vi "string.RemoveIllegalChars.vi"(7 "mode (file)":enum16{"filename", "database", "alphanumeric"}(ring), 8 "error in (no error)":errorcluster, 11 "string in":string) -> (0 "error out":errorcluster, 2 "illegal characters":string, 3 "legal string out":string)   [LabVIEW 2020]
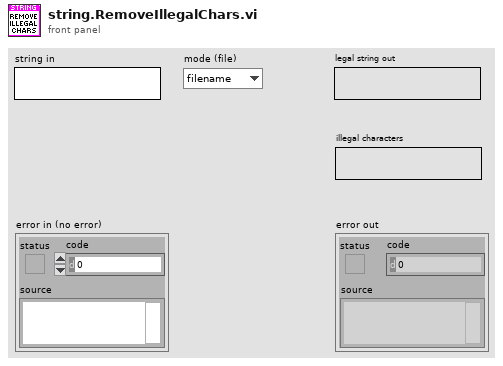
[diagram p1: front panel]
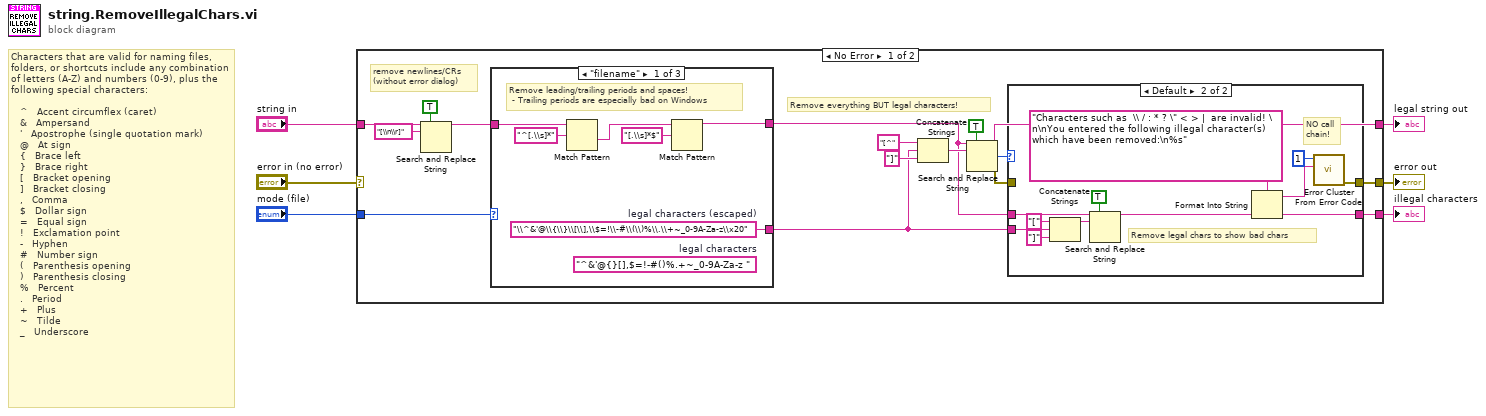
[diagram p0: block diagram]
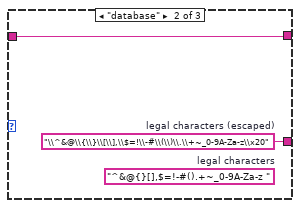
[diagram p2: hidden frame]
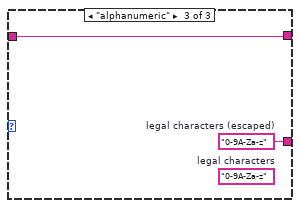
[diagram p3: hidden frame]
diagram:
  # "Characters that are valid for naming files, folders, or shortcuts include any combination of letters (A-Z) and numbers (0-9), plus the following special characters: \n\n   ^   Accent circumflex (caret)\n   &   Ampersand\n   '   Apostrophe (single quotation mark)\n   @   At sign\n   {   Brace left\n   }   Brace right\n   [   Bracket opening\n   ]   Bracket closing\n   ,   Comma\n   $   Dollar sign\n   =   Equal sign\n   !   Exclamation point\n   -   Hyphen\n   #   Number sign\n   (   Parenthesis opening\n   )   Parenthesis closing\n   %   Percent\n   .   Period\n   +   Plus\n   ~   Tilde\n   _   Underscore"
  n1 = case shown="No Error" "error in (no error)" {
    selector: "error in (no error)" -> [_ w45]
    tunnel: "string in" -> [w10 _]
    tunnel: [w21 _] -> w5
    tunnel: [w15 w45] -> w3
    tunnel: [w13 _] -> w2
    tunnel: "mode (file)" -> [w9 _]
    frame No Error {
      # "remove newlines/CRs\n(without error dialog)"
      # "Remove everything BUT legal characters!"
      n2 = Search and Replace String(replace all?=TRUE ("replace all? (F)"), input string=w10, search string="[\\n\\r]") -> (result string=w8:string)  [unwired: 5 in, 3 out]
      n3 = case shown="\"filename\"" w9 {
        tunnel: [w28 w30 w32] -> w17
        tunnel: w8 -> [w27 w29 w31]
        tunnel: [w23 w29 w31] -> w7
        frame "filename" {
          (unwired) "^&'@{}[],$=!-#()%.+~_0-9A-Za-z "  # legal characters
          w28 = "\\^&'@\\{\\}\\[\\],\\$=!\\-#\\(\\)%\\.\\+~_0-9A-Za-z\\x20"  # legal characters (escaped)
          # "Remove leading/trailing periods and spaces! \n - Trailing periods are especially bad on Windows"
          n4 = Match Pattern(string=w27, regular expression="^[.\\s]*") -> (after substring=w24:string)  [unwired: 1 in, 3 out]
          n5 = Match Pattern(string=w24, regular expression="[.\\s]*$") -> (before substring=w23:string)  [unwired: 1 in, 3 out]
        }
        frame "database" {
          (unwired) "^&@{}[],$=!-#().+~_0-9A-Za-z "  # legal characters
          w30 = "\\^&@\\{\\}\\[\\],\\$=!\\-#\\(\\)\\.\\+~_0-9A-Za-z\\x20"  # legal characters (escaped)
        }
        frame "alphanumeric" {
          (unwired) "0-9A-Za-z"  # legal characters
          w32 = "0-9A-Za-z"  # legal characters (escaped)
        }
      }
      n6 = Concatenate Strings("[^" ("string"), w17, "]" ("string")) -> (w20:string)
      n7 = Search and Replace String(replace all?=TRUE ("replace all? (F)"), input string=w7, search string=w20) -> (result string=w21:string, number of replacements=w14:i32, error out=w16:errorcluster)  [unwired: 5 in, 1 out]
      n8 = case shown="Default" w14 {
        tunnel: w17 -> [_ w44]
        tunnel: w16 -> [w33 _]
        tunnel: [w33 w34] -> w15
        tunnel: w7 -> [_ w41]
        tunnel: [_ w37] -> w13
        frame 0 {
          # "No bad chars!"
        }
        frame Default {
          # "NO call\nchain!"
          # "Remove legal chars to show bad chars"
          n9 = Concatenate Strings("[" ("string"), w44, "]" ("string")) -> (w40:string)
          n10 = Search and Replace String(replace all?=TRUE ("replace all? (F)"), input string=w41, search string=w40) -> (result string=w37:string)  [unwired: 5 in, 3 out]
          n11 = Format Into String(format string="Characters such as  \\ / : * ? \" < > |  are invalid! \n\nYou entered the following illegal character(s) which have been removed:\n%s", w37) -> (resulting string=w35:string)  [unwired: 2 in, 1 out]
          n12 = call <vilib>:"Error Cluster From Error Code.vi"("error message (\"\")"=w35, "error code (0)"=1) -> ("error out"=w34:errorcluster)  [unwired: 7 in]
        }
      }
    }
    frame Error {
    }
  }
  "legal string out" <- w5
  "error out" <- w3
  "illegal characters" <- w2
